vi "Write configuration.vi"(8 "error in (no error)":errorcluster, 10 "configuration":refnum<class "CEF_serializable configuration.lvclass">, 11 "Abstract DMM in":refnum<class "DMM Instrument.lvclass">) -> (0 "error out":errorcluster, 3 "Abstract DMM out":refnum<class "DMM Instrument.lvclass">)   [LabVIEW 2025, in "DMM.lvlib" / "DMM Instrument.lvclass"]
uses:
  DMM Instrument.lvclass
  Users/Public/Documents/Sandia National Labs/TSS Plugin/CEF.lvlibp/serializable configuration/CEF_serializable configuration.lvclass
  DMM configuration/DMM configuration.lvclass
  DMM Instrument.lvclass/DMM Instrument.ctl
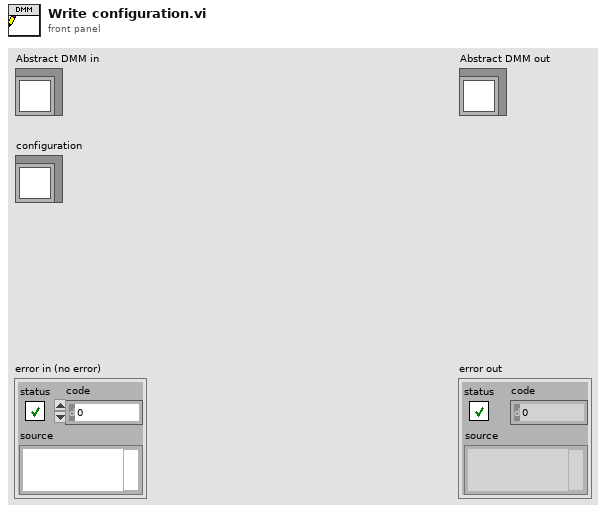
[diagram p1: front panel]
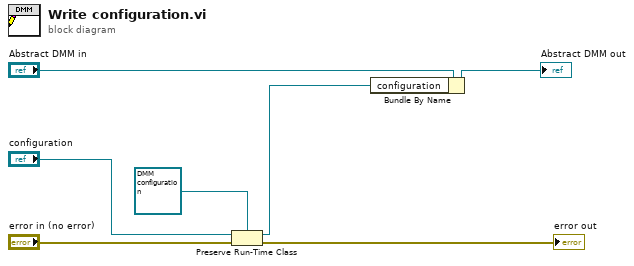
[diagram p0: block diagram]
diagram:
  n1 = Preserve Run-Time Class(object in="configuration", error in="error in (no error)", 2:refnum<class "DMM configuration.lvclass"> refnum ("DMM.lvlib:DMM configuration.lvclass")) -> (object out=w2:refnum<class "DMM configuration.lvclass">, error out=→"error out":errorcluster)
  n2 = Bundle By Name(cluster="Abstract DMM in", "configuration"=w2) -> (→"Abstract DMM out":refnum<class "DMM Instrument.lvclass">)
